vi "http read header.vi"(9 "default value":string, 10 "header field name":string, 11 "headers":T1) -> (1 "found":bool, 3 "value":string)   [LabVIEW 2016, in "Basic HTTP server.lvclass"]
uses:
  Basic HTTP server.lvclass
  http header data.ctl
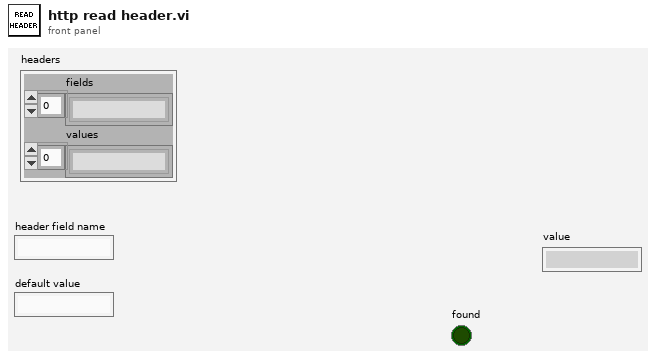
[diagram p1: front panel]
types:
  T1 = typedef "Basic HTTP server.lvclass/http header data.ctl" = cluster{"fields":string[], "values":string[]}
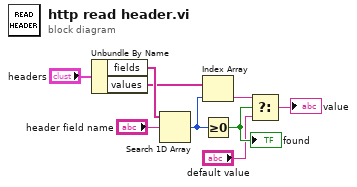
[diagram p0: block diagram]
diagram:
  n1 = Unbundle By Name("headers") -> ("fields"=w8:string[], "values"=w7:string[])
  n2 = Search 1D Array(1D array=w8, element="header field name") -> (index of element=w6:i32)  [unwired: 1 in]
  n3 = Index Array(array=w7, index=w6) -> (element=w4:string)
  n4 = Greater Or Equal To 0?(x=w6) -> (x >= 0?=w5:bool)
  "found" <- w5
  n5 = Select(t=w4, s=w5, f="default value") -> (s? t:f=→"value":string)
